vi "DriftFileHeader.vi"() -> ()   [LabVIEW 2014]
panel:
  in  "End value (V)":sgl min=-10 max=10 format="%#_6p"
  in  "Start value (V)":sgl min=-10 max=10 format="%#_6p"
  in  "End of Sweep":T1 {"Z control time (s)" min=0 max=10 step=0.0001 format="%.3p"; "End settling time (s)" step=0.0001 format="%.3p"}
  in  "Sweep Timing":T2 {"Integration time (s)" min=0 max=20 step=0.0001 format="%.3p"; "Settling time (s)" step=0.0001 format="%.3p"; "Max. slew rate (V/s)" format="%.3p"}
  in  "Initialization":T3 {"Initial settling time (s)" step=0.0001 format="%.3p"; "Z offset (m)" format="%.3p"; "Z averaging time (s)" min=0 max=10 step=0.0001 format="%.3p"}
  in  "Drift Correction":T4
  out "refnum out":refnum<file>
  in  "error in":errorcluster
  in  "file (use dialog)":path
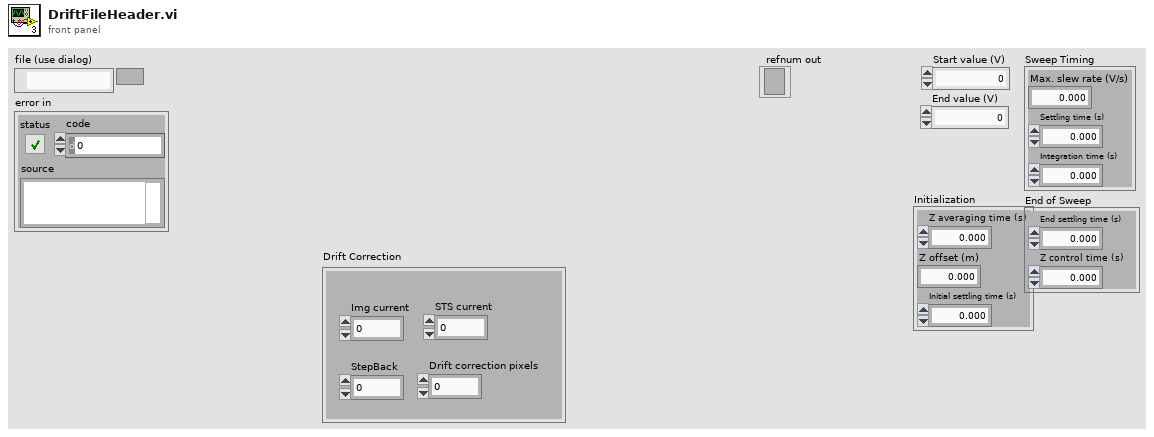
[diagram p1: front panel]
types:
  T1 = cluster{"End settling time (s)":sgl, "Z control time (s)":sgl}
  T2 = cluster{"Max. slew rate (V/s)":sgl, "Settling time (s)":sgl, "Integration time (s)":sgl}
  T3 = cluster{"Z averaging time (s)":sgl, "Z offset (m)":sgl, "Initial settling time (s)":sgl}
  T4 = cluster{"Img current":dbl, "STS current":dbl, "StepBack":dbl, "Drift correction pixels":dbl}
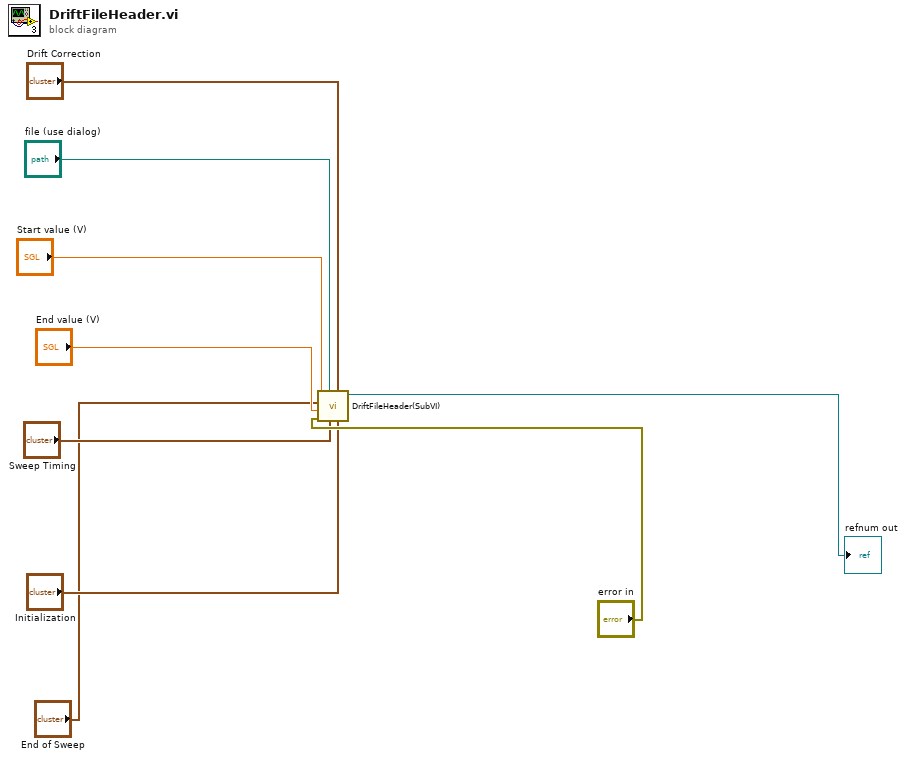
[diagram p0: block diagram]
diagram:
  n1 = call "DriftFileHeader(SubVI).vi"("Initialization"="Initialization", "Drift Correction"="Drift Correction", "Sweep Timing"="Sweep Timing", "file (use dialog)"="file (use dialog)", "error in (no error)"="error in", "End value (V)"="End value (V)", "End of Sweep"="End of Sweep", "Start value (V)"="Start value (V)") -> ("Byte Stream File out"=→"refnum out":refnum<file>)  [unwired: 3 in]
